vi "DECM Get Counter Internal Output.vi"(0 "DAQmx Task In":refnum<k21>, 11 "error in":errorcluster) -> (4 "DAQmx Task Out":refnum<k21>, 8 "Internal Counter Output":tag, 15 "error out":errorcluster)   [LabVIEW 2021, in "DAQ_Digital Edge Count Measurement.lvlib"]
doc: "Returns the internal counter output terminal for the counter choosed in the input counter task"
uses:
  DAQ_Digital Edge Count Measurement.lvlib
  <resource>/objmgr/daqmx.rc
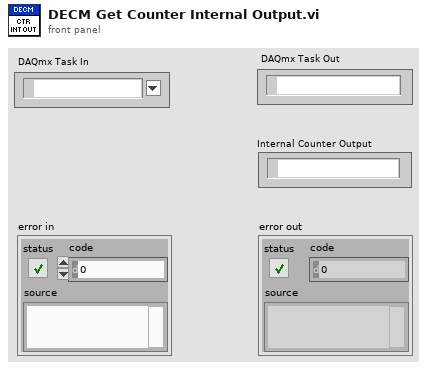
[diagram p1: front panel]
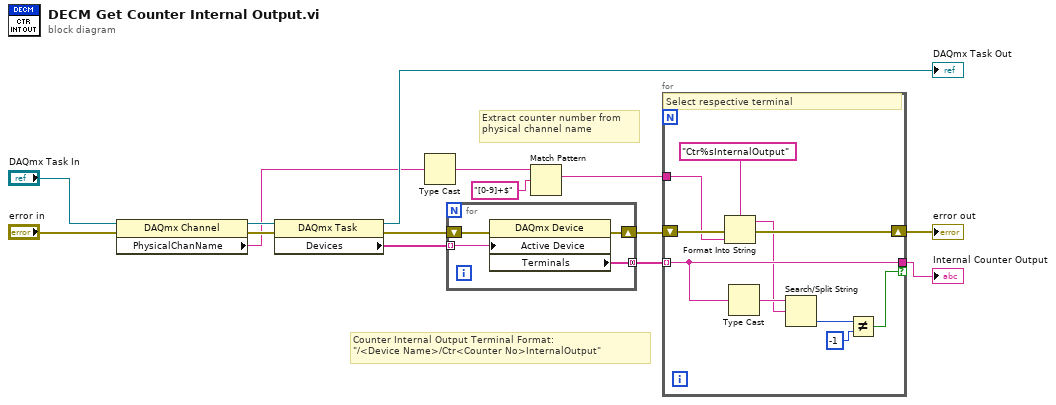
[diagram p0: block diagram]
diagram:
  # "Extract counter number from physical channel name"
  # "Counter Internal Output Terminal Format: \n\"/<Device Name>/Ctr<Counter No>InternalOutput\""
  n1 = property class="DAQmx Channel"(reference="DAQmx Task In", error in="error in") -> (reference out=w9:refnum<k21>, error out=w11:errorcluster, "PhysicalChanName"=w7:tag)
  n2 = property class="DAQmx Task"(reference=w9, error in=w11) -> (reference out=→"DAQmx Task Out":refnum<k21>, error out=w15:errorcluster, "Devices"=w1:tag[])
  n3 = Type Cast(x=w7) -> (*(type *) &x=w8:string)  [unwired: 1 in]
  n4 = for {
    tunnel: [w18] -> w6 mode=concatenating
    shift-right: [w17] -> w4
    shift-left: w15 -> [w19]
    tunnel: w1 -> [w16] mode=indexing
    n5 = property class="DAQmx Device"(error in=w19, "Active Device"=w16) -> (error out=w17:errorcluster, "Terminals"=w18:tag[])  [unwired: 1 in, 1 out]
  }
  n6 = Match Pattern(string=w8, regular expression="[0-9]+$") -> (match substring=w5:string)  [unwired: 1 in, 3 out]
  n7 = for {
    tunnel: w6 -> [w25] mode=indexing
    tunnel: w5 -> [w26]
    shift-right: [w29] -> w3
    shift-left: w4 -> [w28]
    tunnel: [w25] -> w2 if=w20
    # "Select respective terminal"
    n8 = Format Into String(format string="Ctr%sInternalOutput", error in=w28, w26) -> (resulting string=w23:string, error out=w29:errorcluster)  [unwired: 1 in]
    n9 = Type Cast(x=w25) -> (*(type *) &x=w24:string)  [unwired: 1 in]
    n10 = Search/Split String(string=w24, search string/char (-)=w23) -> (offset of match=w22:i32)  [unwired: 1 in, 2 out]
    n11 = Not Equal?(x=w22, y=-1) -> (x != y?=w20:bool)
  }
  "error out" <- w3
  "Internal Counter Output" <- w2
